vi "营养盐读取平行样数据.vi"(8 "error in (no error)":errorcluster, 10 "站号":u16(ring)=1 items=["总磷"=1, "总氮"=2, "氨氮"=3, "CODMn"=21, "CODCr"=22], 11 "MB session in":refnum<class "MB_Master.lvclass">) -> (0 "error out":errorcluster, 3 "测量数据区":T1)   [LabVIEW 2016, in "质控单元V4.lvlib"]
uses:
  <vilib>/Plasmionique/MB Master/MB_Master/MB_Master.lvclass
  <vilib>/Plasmionique/MB Master/MB Master.lvlib
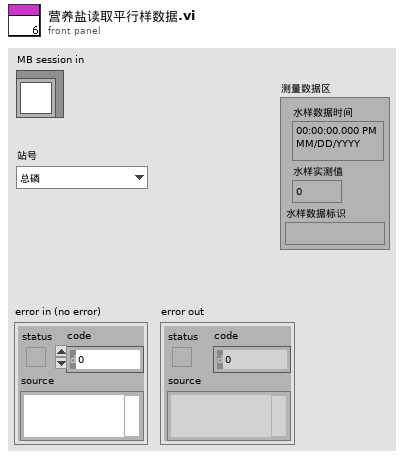
[diagram p1: front panel]
types:
  T1 = cluster{"水样数据时间":timestamp, "水样实测值":sgl, "水样数据标识":string}
  T2 = cluster{"time stamp":timestamp, "数值":sgl, "string":string}
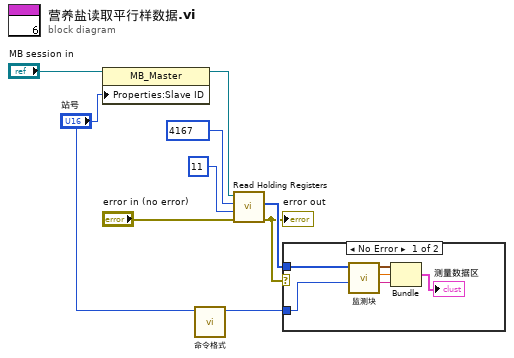
[diagram p0: block diagram]
diagram:
  n1 = property class="MB_Master"(reference="MB session in", "Properties:Slave ID"="站号") -> (reference out=w6:refnum<class "MB_Master.lvclass">)  [unwired: 1 in, 1 out]
  n2 = call "命令格式.vi"("站号"="站号") -> ("命令格式"=w1:u16)  [unwired: 10 in]
  n3 = call <vilib>:"Read Holding Registers.vi"("error in (no error)"="error in (no error)", "quantity"=u16 11, "starting address"=u16 4167, "MB session in"=w6) -> ("error out"=w3:errorcluster, "Registers"=w4:u16[])  [unwired: 5 in, 1 out]
  "error out" <- w3
  n4 = case shown="No Error" w3 {
    tunnel: w4 -> [w15 _]
    tunnel: w1 -> [w10 _]
    frame No Error {
      n5 = call "监测块.vi"("命令格式"=w10, "数组"=w15) -> ("string"=w12:string, "数值"=w13:sgl, "time stamp"=w14:timestamp)  [unwired: 7 in]
      n6 = Bundle("time stamp"=w14, "数值"=w13, "string"=w12) -> (→"测量数据区":T2)  [unwired: 1 in]
    }
    frame Error {
    }
  }
